vi "升立德IO读写Main.vi"(6 "结果":bool, 8 "error in":errorcluster caption="错误输入（无错误）", 9 "IO输出":T2, 10 "选择相机":enum16{"相机1", "相机2", "相机3", "相机4"}(ring), 11 "选项":T4=enum."读信号(16bit)") -> (0 "error out":errorcluster caption="错误输出", 1 "触发上升沿":T1, 2 "IO输入":T3, 3 "结果":bool, 4 "IO输出":T2)   [LabVIEW 2014]
uses:
  IOinput.ctl
  IOoutput.ctl
  Controls/MsgAction.ctl
panel:
  out "收到触发信号次数第一次收到触发信号不动作":i32
  out "触发信号":bool[](array[boolean])
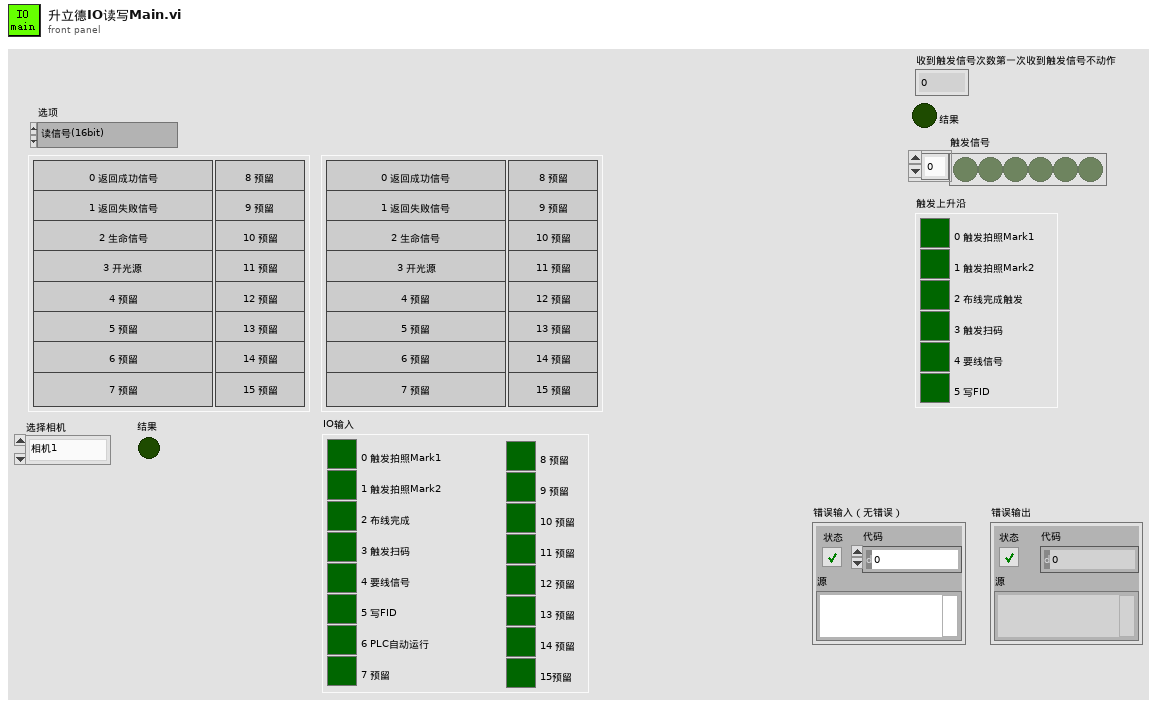
[diagram p1: front panel]
types:
  T1 = typedef "触发上升沿.ctl" = cluster{"0 触发拍照Mark1":bool, "1 触发拍照Mark2":bool, "2 布线完成触发":bool, "3 触发扫码":bool, "4 要线信号":bool, "5 写FID":bool}
  T2 = typedef "IOoutput.ctl" = cluster{"0 返回成功信号":bool, "1 返回失败信号":bool, "2 生命信号":bool, "3 开光源":bool, "4 预留":bool, "5 预留":bool, "6 预留":bool, "7 预留":bool, "8 预留":bool, "9 预留":bool, "10 预留":bool, "11 预留":bool, "12 预留":bool, "13 预留":bool, "14 预留":bool, "15 预留":bool}
  T3 = typedef "IOinput.ctl" = cluster{"0 触发拍照Mark1":bool, "1 触发拍照Mark2":bool, "2 布线完成":bool, "3 触发扫码":bool, "4 要线信号":bool, "5 写FID":bool, "6 PLC自动运行":bool, "7 预留":bool, "8 预留":bool, "9 预留":bool, "10 预留":bool, "11 预留":bool, "12 预留":bool, "13 预留":bool, "14 预留":bool, "15预留":bool}
  T4 = typedef "升立德IOAction.ctl" = enum16{"IO卡初始化", "读信号(16bit)", "写信号(16bit)", "开光源", "写成功/失败信号ON", "写成功&&失败信号OFF", "写失败信号ON", "写失败信号OFF", "写生命信号", "GetInfo", "清除目标"}
  T5 = typedef "MsgAction.ctl" = enum16{"初始化", "添加消息", "区分结果添加消息", "清空消息", "获取消息"}
  T6 = cluster{"Boolean array[0]":bool, "Boolean array[1]":bool, "Boolean array[2]":bool, "Boolean array[3]":bool, "Boolean array[4]":bool, "Boolean array[5]":bool, "Boolean array[6]":bool, "Boolean array[7]":bool, "Boolean array[8]":bool, "Boolean array[9]":bool, "Boolean array[10]":bool, "Boolean array[11]":bool, "Boolean array[12]":bool, "Boolean array[13]":bool, "Boolean array[14]":bool, "Boolean array[15]":bool}
  T7 = cluster{"[0]":bool, "[1]":bool, "[2]":bool, "[3]":bool, "[4]":bool, "[5]":bool}
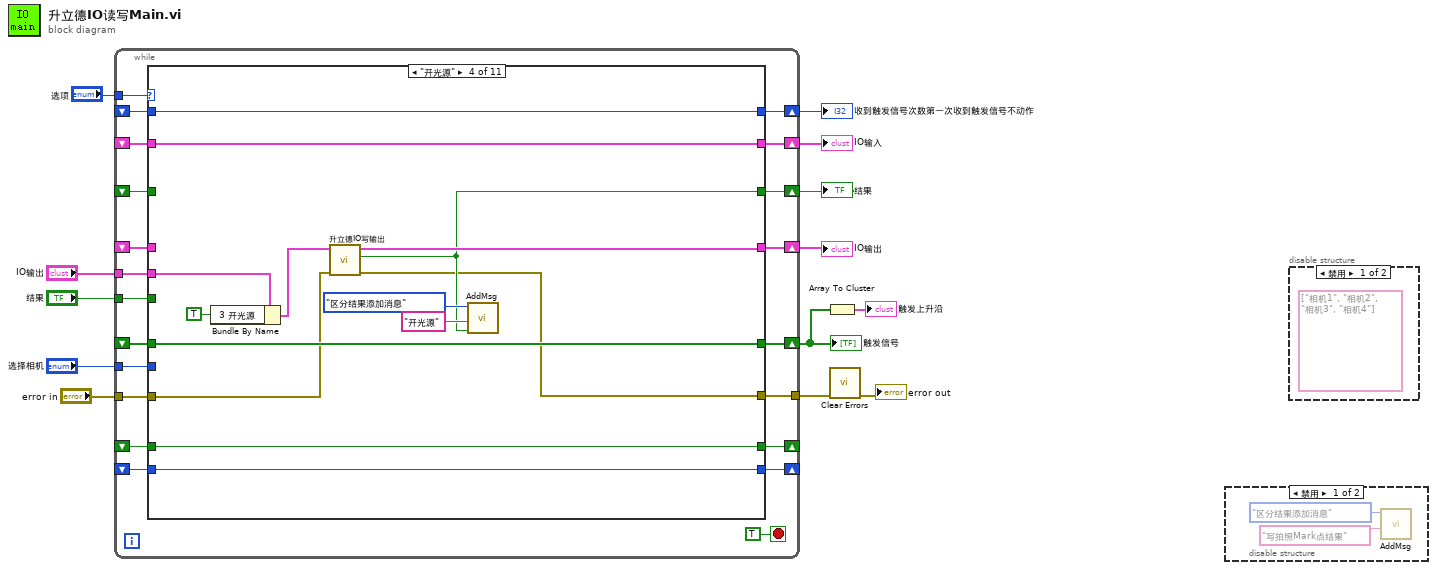
[diagram p0: block diagram]
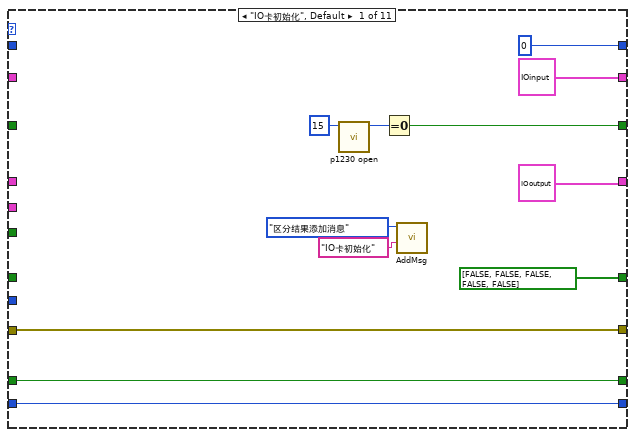
[diagram p4: hidden frame]
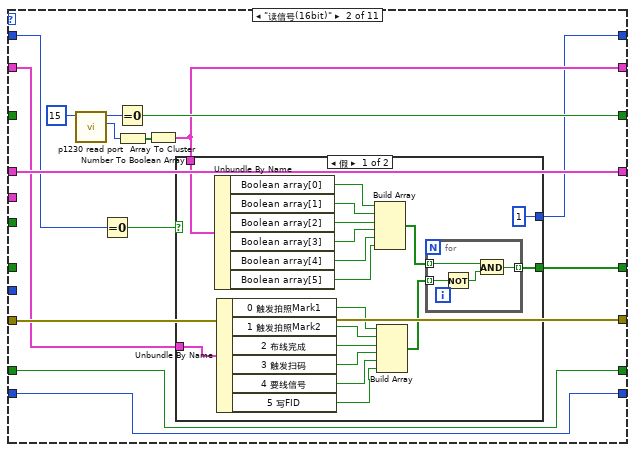
[diagram p5: hidden frame]
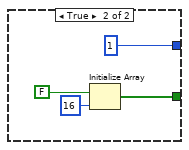
[diagram p6: hidden frame]
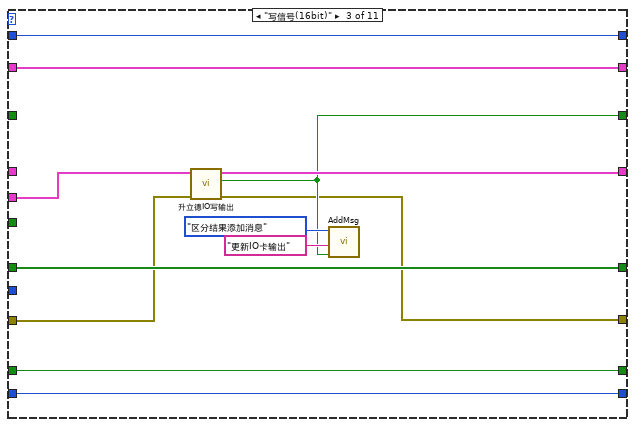
[diagram p7: hidden frame]
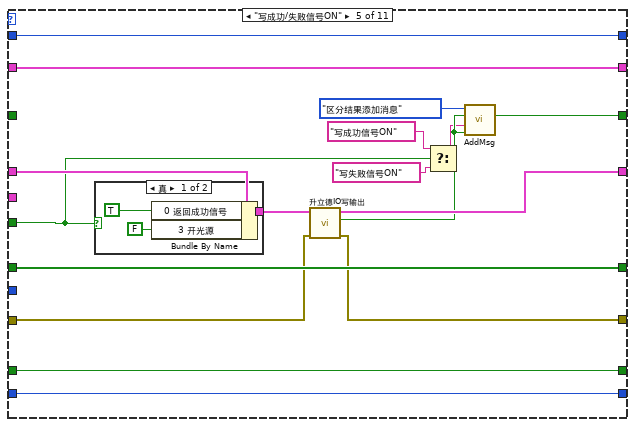
[diagram p8: hidden frame]
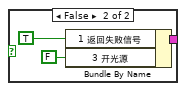
[diagram p9: hidden frame]
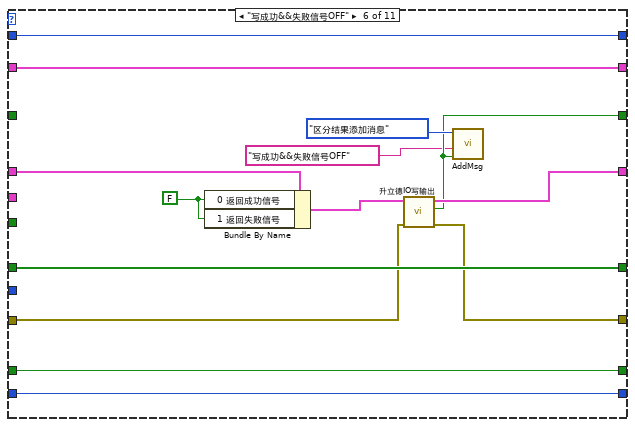
[diagram p10: hidden frame]
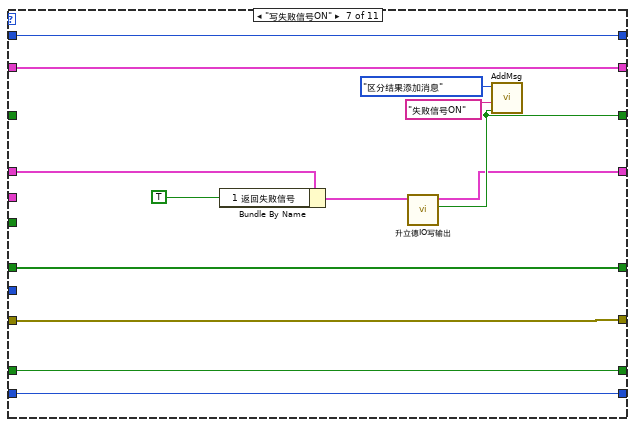
[diagram p11: hidden frame]
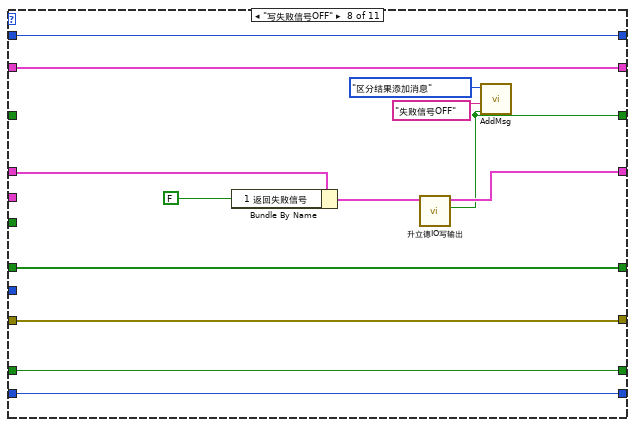
[diagram p12: hidden frame]
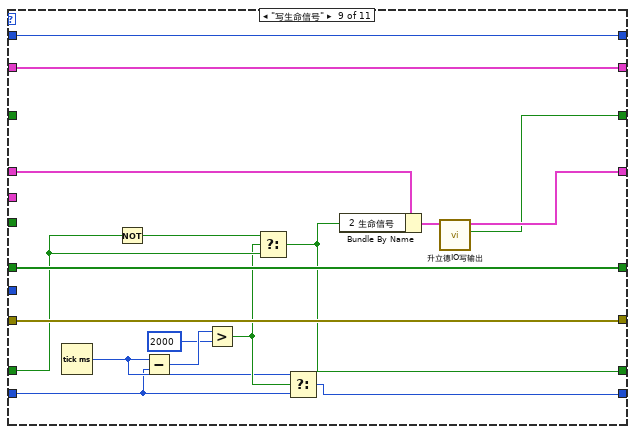
[diagram p13: hidden frame]
diagram:
  n1 = while {
    tunnel: "选项" -> [w33]
    tunnel: [w32] -> w8
    tunnel: "error in" -> [w31]
    shift-right: [w30] -> w11
    shift-left: _ -> [w29]
    shift-right: [w27] -> w9
    shift-left: _ -> [w26]
    tunnel: "IO输出" -> [w25]
    tunnel: "结果" -> [w24]
    shift-right: [w23] -> w6
    shift-left: _ -> [w22]
    shift-right: [w28] -> w3
    shift-left: _ -> [w21]
    tunnel: "选择相机" -> [w20]
    shift-right: [w19] -> w1
    shift-left: _ -> [w18]
    shift-right: [w15] -> _
    shift-left: _ -> [w16]
    shift-right: [w14] -> _
    shift-left: _ -> [w17]
    stop <- TRUE stop-if-true
    n2 = case shown="\"开光源\"" w33 {
      tunnel: [w46 w61 w90 w105 w120 w141 w163 w170 w192 w201 w208] -> w32
      tunnel: w31 -> [w46 w61 w95 w110 w121 w142 w163 w170 w192 w201 w208]
      tunnel: [T3 {"0 触发拍照Mark1"=FALSE, "1 触发拍照Mark2"=FALSE, "2 布线完成"=FALSE, "3 触发扫码"=FALSE, "4 要线信号"=FALSE, "5 写FID"=FALSE, "6 PLC自动运行"=FALSE, "7 预留"=FALSE, "8 预留"=FALSE, "9 预留"=FALSE, "10 预留"=FALSE, "11 预留"=FALSE, "12 预留"=FALSE, "13 预留"=FALSE, "14 预留"=FALSE, "15预留"=FALSE} ("IO输入") w54 w93 w108 w123 w147 w158 w171 w190 w202 w210] -> w30
      tunnel: w29 -> [_ w52 w93 w108 w123 w147 w158 w171 w190 w202 w210]
      tunnel: [bool[] [FALSE, FALSE, FALSE, FALSE, FALSE] w60 w97 w111 w126 w148 w159 w169 w191 w198 w205] -> w28
      tunnel: [T2 {"0 返回成功信号"=FALSE, "1 返回失败信号"=FALSE, "2 生命信号"=FALSE, "3 开光源"=FALSE, "4 预留"=FALSE, "5 预留"=FALSE, "6 预留"=FALSE, "7 预留"=FALSE, "8 预留"=FALSE, "9 预留"=FALSE, "10 预留"=FALSE, "11 预留"=FALSE, "12 预留"=FALSE, "13 预留"=FALSE, "14 预留"=FALSE, "15 预留"=FALSE} ("IO输出") w53 w94 w109 w129 w150 w157 w172 w189 w200 w209] -> w27
      tunnel: w26 -> [_ w53 _ _ w125 w146 w164 w173 w193 w200 w209]
      tunnel: w25 -> [_ _ w96 w102 _ _ _ _ _ _ _]
      tunnel: w24 -> [_ _ _ _ w117 _ _ _ _ _ _]
      tunnel: [w38 w58 w92 w107 w127 w149 w161 w168 w188 w199 w207] -> w23
      tunnel: w22 -> [_ _ _ _ _ _ _ _ _ w199 w207]
      tunnel: w21 -> [_ _ w97 w111 w126 w148 w159 w169 w191 w198 w205]
      tunnel: w20 -> [_ _ _ _ _ _ _ _ _ _ _]
      tunnel: [0 w49 w91 w106 w122 w143 w154 w167 w187 w197 w206] -> w19
      tunnel: w18 -> [_ w51 w91 w106 w122 w143 w154 w167 w187 w197 w206]
      tunnel: w17 -> [w35 w47 w88 w103 w118 w139 w152 w165 w179 w195 w203]
      tunnel: w16 -> [w36 w48 w89 w104 w119 w140 w153 w166 w184 w196 w204]
      tunnel: [w36 w48 w89 w104 w119 w140 w153 w166 w182 w196 w204] -> w15
      tunnel: [w35 w47 w88 w103 w118 w139 w152 w165 w178 w195 w203] -> w14
      frame "IO卡初始化", Default {
        n3 = call "p1230 open.vi"("board_id"=u32 15) -> ("function return"=w41:u32)  [unwired: 9 in, 1 out]
        n4 = Equal To 0?(x=w41) -> (x = 0?=w38:bool)
        n5 = call "AddMsg.vi"("添加消息"="IO卡初始化" ("消息显示"), "消息Action"=MsgAction."区分结果添加消息") -> ()  [unwired: 2 in, 1 out]
      }
      frame "读信号(16bit)" {
        n6 = call "p1230 read port.vi"("board_id"=u32 15) -> ("pData out"=w56:u32, "function return"=w57:u32)  [unwired: 8 in, 1 out]
        n7 = Equal To 0?(x=w51) -> (x = 0?=w50:bool)
        n8 = Equal To 0?(x=w57) -> (x = 0?=w58:bool)
        n9 = Number To Boolean Array(number=w56) -> (Boolean array=w55:bool[])
        n10 = Array To Cluster(array=w55) -> (cluster=w54:T6)
        n11 = case shown="假" w50 {
          tunnel: [w79 w85] -> w60
          tunnel: w54 -> [w72 _]
          tunnel: w52 -> [w66 _]
          tunnel: [1 1] -> w49
          frame False {
            n12 = Unbundle By Name(w72) -> ("Boolean array[0]"=w78:bool, "Boolean array[1]"=w77:bool, "Boolean array[2]"=w76:bool, "Boolean array[3]"=w75:bool, "Boolean array[4]"=w74:bool, "Boolean array[5]"=w63:bool)
            n13 = Unbundle By Name(w66) -> ("0 触发拍照Mark1"=w67:bool, "1 触发拍照Mark2"=w68:bool, "2 布线完成"=w69:bool, "3 触发扫码"=w70:bool, "4 要线信号"=w71:bool, "5 写FID"=w62:bool)
            n14 = Build Array(w78, w77, w76, w75, w74, w63) -> (w73:bool[])
            n15 = Build Array(w67, w68, w69, w70, w71, w62) -> (w65:bool[])
            n16 = for {
              tunnel: [w80] -> w79 mode=indexing
              tunnel: w73 -> [w81] mode=indexing
              tunnel: w65 -> [w83] mode=indexing
              n17 = Not(x=w83) -> (.not. x?=w82:bool)
              n18 = And(x=w81, y=w82) -> (x .and. y?=w80:bool)
            }
          }
          frame True {
            n19 = Initialize Array(FALSE, 16 ("维数大小")) -> (w85:bool[])
          }
        }
      }
      frame "写信号(16bit)" {
        n20 = call "升立德IO写输出.vi"("IO输出"=w96, "error in (no error)"=w95) -> ("IO输出"=w94:T2, "结果"=w92:bool, "error out"=w90:errorcluster)  [unwired: 5 in]
        n21 = call "AddMsg.vi"("Result"=w92, "添加消息"="更新IO卡输出", "消息Action"=MsgAction."区分结果添加消息") -> ()  [unwired: 1 in, 1 out]
      }
      frame "开光源" {
        n22 = Bundle By Name(cluster=w102, "3 开光源"=TRUE) -> (w100:T2)
        n23 = call "升立德IO写输出.vi"("IO输出"=w100, "error in (no error)"=w110) -> ("IO输出"=w109:T2, "结果"=w107:bool, "error out"=w105:errorcluster)  [unwired: 5 in]
        n24 = call "AddMsg.vi"("Result"=w107, "添加消息"="开光源", "消息Action"=MsgAction."区分结果添加消息") -> ()  [unwired: 1 in, 1 out]
      }
      frame "写成功/失败信号ON" {
        n25 = case shown="真" w117 {
          tunnel: w125 -> [w133 w137]
          tunnel: [w132 w136] -> w124
          frame True {
            n26 = Bundle By Name(cluster=w133, "0 返回成功信号"=TRUE ("拍照结果"), "3 开光源"=FALSE ("3 预留")) -> (w132:T2)
          }
          frame False {
            n27 = Bundle By Name(cluster=w137, "1 返回失败信号"=TRUE ("拍照结果"), "3 开光源"=FALSE ("3 预留")) -> (w136:T2)
          }
        }
        n28 = call "升立德IO写输出.vi"("IO输出"=w124, "error in (no error)"=w121) -> ("IO输出"=w129:T2, "结果"=w127:bool, "error out"=w120:errorcluster)  [unwired: 5 in]
        n29 = Select(t="写成功信号ON" ("添加消息"), s=w117, f="写失败信号ON" ("添加消息")) -> (s? t:f=w114:string)
        n30 = call "AddMsg.vi"("Result"=w127, "添加消息"=w114, "消息Action"=MsgAction."区分结果添加消息") -> ()  [unwired: 1 in, 1 out]
      }
      frame "写成功&&失败信号OFF" {
        w138 = FALSE ("拍照结果")
        n31 = Bundle By Name(cluster=w146, "0 返回成功信号"=w138, "1 返回失败信号"=w138) -> (w145:T2)
        n32 = call "升立德IO写输出.vi"("IO输出"=w145, "error in (no error)"=w142) -> ("IO输出"=w150:T2, "结果"=w149:bool, "error out"=w141:errorcluster)  [unwired: 5 in]
        n33 = call "AddMsg.vi"("Result"=w149, "添加消息"="写成功&&失败信号OFF", "消息Action"=MsgAction."区分结果添加消息") -> ()  [unwired: 1 in, 1 out]
      }
      frame "写失败信号ON" {
        n34 = Bundle By Name(cluster=w164, "1 返回失败信号"=TRUE ("5 拍照Mark/PCB孔图像处理OK")) -> (w160:T2)
        n35 = call "升立德IO写输出.vi"("IO输出"=w160) -> ("IO输出"=w157:T2, "结果"=w161:bool)  [unwired: 6 in, 1 out]
        n36 = call "AddMsg.vi"("Result"=w161, "添加消息"="失败信号ON", "消息Action"=MsgAction."区分结果添加消息") -> ()  [unwired: 1 in, 1 out]
      }
      frame "写失败信号OFF" {
        n37 = Bundle By Name(cluster=w173, "1 返回失败信号"=FALSE ("5 拍照Mark/PCB孔图像处理OK")) -> (w176:T2)
        n38 = call "升立德IO写输出.vi"("IO输出"=w176) -> ("IO输出"=w172:T2, "结果"=w168:bool)  [unwired: 6 in, 1 out]
        n39 = call "AddMsg.vi"("Result"=w168, "添加消息"="失败信号OFF", "消息Action"=MsgAction."区分结果添加消息") -> ()  [unwired: 1 in, 1 out]
      }
      frame "写生命信号" {
        n40 = Tick Count (ms)() -> (millisecond timer value=w180:u32)
        n41 = Not(x=w184) -> (.not. x?=w183:bool)
        n42 = Subtract(x=w180, y=w179) -> (x-y=w186:u32)
        n43 = Greater?(x=w186, y=u32 2000) -> (0:w181:bool)
        n44 = Select(t=w183, s=w181, f=w184) -> (s? t:f=w182:bool)
        n45 = Select(t=w180, s=w181, f=w179) -> (s? t:f=w178:u32)
        n46 = Bundle By Name(cluster=w193, "2 生命信号"=w182) -> (w194:T2)
        n47 = call "升立德IO写输出.vi"("IO输出"=w194) -> ("IO输出"=w189:T2, "结果"=w188:bool)  [unwired: 6 in, 1 out]
      }
      frame "GetInfo" {
      }
      frame "清除目标" {
      }
    }
  }
  "IO输入" <- w11
  "IO输出" <- w9
  "结果" <- w6
  "触发信号" <- w3
  "收到触发信号次数第一次收到触发信号不动作" <- w1
  n48 = Array To Cluster(array=w3) -> (cluster=→"触发上升沿":T7)
  n49 = call <vilib>:"Clear Errors.vi"("error in (no error)"=w8) -> ("error out"=→"error out":errorcluster)  [unwired: 5 in, 1 out]
  n50 = disable-structure shown="禁用" {
    frame Disabled {
      n51 = call "AddMsg.vi"("添加消息"="写拍照Mark点结果", "消息Action"=MsgAction."区分结果添加消息") -> ()  [unwired: 2 in, 1 out]
    }
    frame Enabled {
    }
  }
  n52 = disable-structure shown="禁用" {
    frame Disabled {
      (unwired) string[] ["相机1", "相机2", "相机3", "相机4"]
    }
    frame Enabled {
    }
  }
